vi "PicoScope5000aSetEtsTimeBuffer.vi"(8 "error in (no error)":errorcluster, 10 "bufferLth":i32, 11 "handle in":i16) -> (0 "error out":errorcluster, 2 "EtsTimeValues":i64[](array[numeric]), 3 "handle out":i16)   [LabVIEW 2009]
doc: "Calls SetEtsTimeBuffer"
uses:
  ps5000a.dll
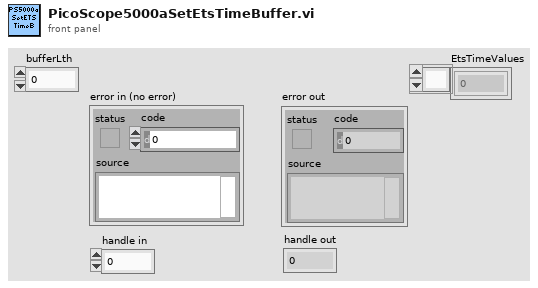
[diagram p1: front panel]
types:
  T1 = enum16{"U8", "I8", "U16", "I16", "U32", "I32", "U64", "I64"}
  T2 = cluster{"status":bool, "code":u32, "source":string}
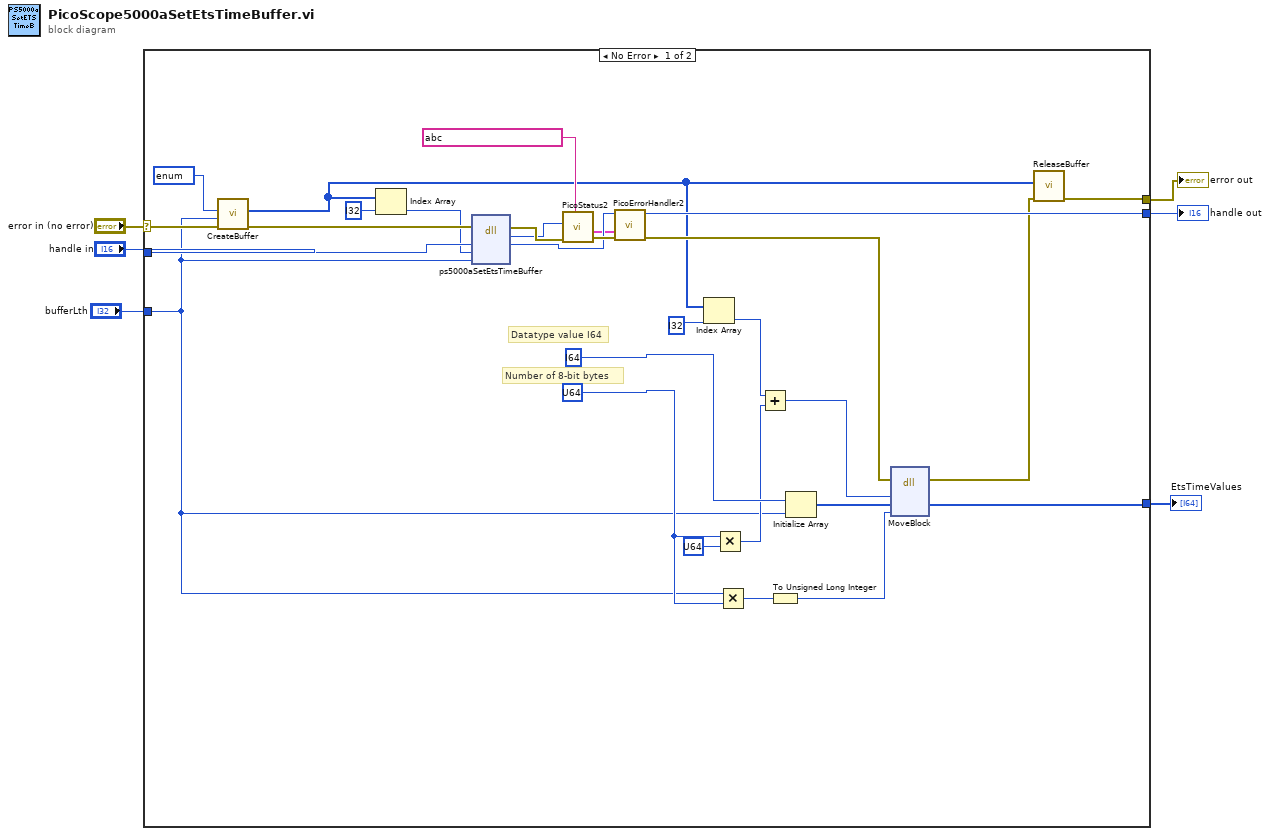
[diagram p0: block diagram]
diagram:
  n1 = case shown="No Error" "error in (no error)" {
    selector: "error in (no error)" -> [w28 w36]
    tunnel: [w26 w36] -> w4
    tunnel: "handle in" -> [w32 w35]
    tunnel: [w29 w35] -> w5
    tunnel: "bufferLth" -> [w10 _]
    tunnel: [w12 _] -> w1
    frame #0 {
      w20 = u64 ? ("y")
      # "Number of 8-bit bytes"
      # "Datatype value I64"
      n2 = call "CreateBuffer.vi"("error in (no error)"=w28, "Buffer size"=w10, "Data type"=T1 ?) -> ("error out"=w27:errorcluster, "Pointer and BufferSize"=w9:u64[])  [unwired: 7 in]
      n3 = Index Array(array=w9, index=i32 ?) -> (element=w25:u64)
      n4 = dll-call lib="ps5000a.dll" fn="ps5000aSetEtsTimeBuffer" ("ps3000.dll:_ps3000_open_unit@0")(error in=w27, "handle"=w32, "buffer"=w25, "bufferLth"=w10) -> (error out=w31:errorcluster, "PICO_STATUS"=w30:u32, "handle"=w29:i16)  [unwired: 4 in, 1 out]
      n5 = call "PicoStatus2.vi"("PICO source"=string ? ("source"), "Error in"=w31, "PICO STATUS"=w30) -> ("error out"=w34:errorcluster, "PICO_STATUS out"=w7:T2)  [unwired: 5 in]
      n6 = call "PicoErrorHandler2.vi"("error in (no error)"=w34, "PICO_STATUS in"=w7, "handle In"=w29) -> ("error out"=w13:errorcluster)  [unwired: 8 in]
      n7 = Index Array(array=w9, index=i32 ?) -> (element=w22:u64)
      n8 = Multiply(x=w20, y=u64 ?) -> (x*y=w21:u64)
      n9 = Multiply(x=w10, y=w20) -> (x*y=w19:u64)
      n10 = Add(x=w22, y=w21) -> (x+y=w18:u64)
      n11 = To Unsigned Long Integer(number=w19) -> (unsigned 32bit integer=w16:u32)
      n12 = Initialize Array(i64 ? ("element"), w10) -> (w17:i64[])
      n13 = dll-call lib="LabVIEW" fn="MoveBlock"(error in=w13, "Source"=w18, "Destination"=w17, "Size"=w16) -> (error out=w14:errorcluster, "Destination"=w12:i64[])  [unwired: 5 in, 1 out]
      n14 = call "ReleaseBuffer.vi"("error in (no error)"=w14, "Pointer and BufferSize"=w9) -> ("error out"=w26:errorcluster)  [unwired: 9 in]
    }
    frame #1 {
    }
  }
  "error out" <- w4
  "handle out" <- w5
  "EtsTimeValues" <- w1
